vi "Arrange Channel List Per-Site.vi"(0 "Channel List String":string, 5 "Site List String":string) -> (4 "Channel List Array":string[](array[string]), 6 "Site List Array":string[](array[string]), 8 "Site Numbers":i32[](array[numeric]))   [LabVIEW 2019]
uses:
  Trim Whitespace [Inlined].vi
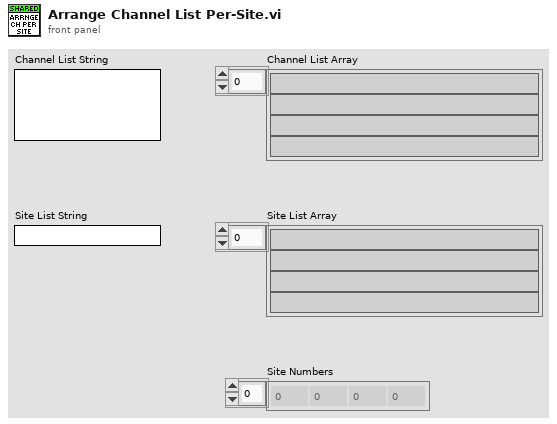
[diagram p1: front panel]
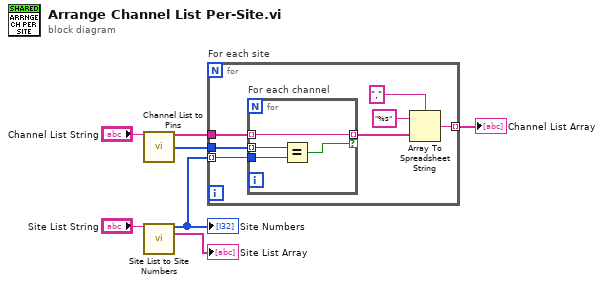
[diagram p0: block diagram]
diagram:
  n1 = call "Channel List to Pins.vi"("Channel List"="Channel List String") -> ("Sites and Pins"=w3:string[], "Sites"=w2:i32[])  [unwired: 12 in, 1 out]
  n2 = call "Site List to Site Numbers.vi"("Site List"="Site List String") -> ("Site Numbers"=w1:i32[], "Sites"=→"Site List Array":string[])  [unwired: 13 in]
  "Site Numbers" <- w1
  n3 = for "For each site" {
    tunnel: w3 -> [w14]
    tunnel: [w10] -> w7 mode=indexing
    tunnel: w2 -> [w9]
    tunnel: w1 -> [w8] mode=indexing
    n4 = for "For each channel" {
      tunnel: w14 -> [w18] mode=indexing
      tunnel: [w18] -> w13 mode=indexing if=w15
      tunnel: w9 -> [w17] mode=indexing
      tunnel: w8 -> [w16]
      n5 = Equal?(x=w17, y=w16) -> (x = y?=w15:bool)
    }
    n6 = Array To Spreadsheet String(delimiter (Tab)=",", array=w13, 3:"%s" ("format string")) -> (spreadsheet string=w10:string)
  }
  "Channel List Array" <- w7
